vi "Universal I-V.vi"() -> ()   [LabVIEW 2021]
panel:
  in  "Tab Control 2":enum32{"V1 vs I", "V2 vs I", "V3 vs I"}(tab)=enum."V2 vs I"
  out "XY Graph":cluster{"Y":dbl[], "Y":dbl[]}[](graph)=[{"Y"=[-1.0, -0.95, -0.9, -0.85, -0.8, -0.75, -0.7, -0.6499999999999999, -0.6, -0.55, -0.5, -0.44999999999999996, -0.3999999999999999, -0.35, -0.29999999999999993, -0.25, -0.19999999999999996, -0.1499999999999999, -0.09999999999999998, -0.04999999999999993, 0.0, 0.050000000000000044, 0.10000000000000009, 0.15000000000000013, 0.20000000000000018, 0.25, 0.30000000000000004, 0.3500000000000001, 0.40000000000000013, 0.4500000000000002, 0.5, 0.55, 0.6000000000000001, 0.6500000000000001, 0.7000000000000002, 0.75, 0.8, 0.8500000000000001, 0.9000000000000001, 0.9500000000000002, 1.0, 0.9499999999999997, 0.8999999999999999, 0.8500000000000001, 0.7999999999999998, 0.75, 0.6999999999999997, 0.6499999999999999, 0.5999999999999996, 0.5499999999999998, 0.5, 0.44999999999999973, 0.3999999999999999, 0.34999999999999964, 0.2999999999999998, 0.25, 0.19999999999999973, 0.1499999999999999, 0.09999999999999964, 0.04999999999999982, 0.0, -0.050000000000000266, -0.10000000000000009, -0.15000000000000036, -0.20000000000000018, -0.25, -0.30000000000000027, -0.3500000000000001, -0.40000000000000036, -0.4500000000000002, -0.5, -0.5500000000000003, -0.6000000000000001, -0.6500000000000004, -0.7000000000000002, -0.75, -0.8000000000000003, -0.8500000000000001, -0.9000000000000004, -0.9500000000000002, -1.0], "Y"=[-1.043934004639324, -0.9887925352579463, -0.9337434547255242, -0.8776183272811331, -0.82231690582607, -0.766602837334161, -0.7120604287683167, -0.6565192233796591, -0.6008463731439775, -0.5453454129858952, -0.49006848731381447, -0.4342878186943741, -0.37878107527949273, -0.3237800120154516, -0.2679185581761966, -0.213113202761182, -0.15731677133399102, -0.10218502786401004, -0.046651896362743354, 0.00868166875831078, 0.06396663101585874, 0.11957605302530742, 0.1754465244847772, 0.23063460766105412, 0.2855722696490664, 0.3412534850248921, 0.3972359875159429, 0.4523442615679825, 0.5071052297686396, 0.5630385018551626, 0.618492497279927, 0.6741412394437152, 0.7295823751559891, 0.7846829671519501, 0.8402139260072709, 0.8957539073517712, 0.9509082828151478, 1.006347213884267, 1.0618881933858204, 1.117535728296589, 1.1727142914289796, 1.1176483875247343, 1.06164806834701, 1.006077475634131, 0.9510367142452216, 0.8955137824533387, 0.840085172731705, 0.7849945500084466, 0.7292096345678497, 0.6733065967707881, 0.6182922860635163, 0.562991828830372, 0.5072925656102947, 0.4519161573664326, 0.39629383647669314, 0.3412476911337492, 0.28535017053922246, 0.23016884332060678, 0.174690100070839, 0.1194653253729142, 0.06376416679748173, 0.008442831801321127, -0.046625501982918545, -0.10205659667499047, -0.15755560828214077, -0.2133671681974733, -0.2683102894086483, -0.3239593006796162, -0.37933857613562044, -0.4349676350135405, -0.49032180903465616, -0.5456061380270941, -0.6007304953378655, -0.656422336649383, -0.7119126845425408, -0.7676135495978567, -0.8227199032513759, -0.8778352764025348, -0.9336491430031517, -0.9893680621687002, -1.0442929042963138]}]
  out "XY Graph 2":cluster{"Y":dbl[], "Y":dbl[]}[](graph)=[{"Y"=[-1.0, -0.95, -0.9, -0.85, -0.8, -0.75, -0.7, -0.6499999999999999, -0.6, -0.55, -0.5, -0.44999999999999996, -0.3999999999999999, -0.35, -0.29999999999999993, -0.25, -0.19999999999999996, -0.1499999999999999, -0.09999999999999998, -0.04999999999999993, 0.0, 0.050000000000000044, 0.10000000000000009, 0.15000000000000013, 0.20000000000000018, 0.25, 0.30000000000000004, 0.3500000000000001, 0.40000000000000013, 0.4500000000000002, 0.5, 0.55, 0.6000000000000001, 0.6500000000000001, 0.7000000000000002, 0.75, 0.8, 0.8500000000000001, 0.9000000000000001, 0.9500000000000002, 1.0, 0.9499999999999997, 0.8999999999999999, 0.8500000000000001, 0.7999999999999998, 0.75, 0.6999999999999997, 0.6499999999999999, 0.5999999999999996, 0.5499999999999998, 0.5, 0.44999999999999973, 0.3999999999999999, 0.34999999999999964, 0.2999999999999998, 0.25, 0.19999999999999973, 0.1499999999999999, 0.09999999999999964, 0.04999999999999982, 0.0, -0.050000000000000266, -0.10000000000000009, -0.15000000000000036, -0.20000000000000018, -0.25, -0.30000000000000027, -0.3500000000000001, -0.40000000000000036, -0.4500000000000002, -0.5, -0.5500000000000003, -0.6000000000000001, -0.6500000000000004, -0.7000000000000002, -0.75, -0.8000000000000003, -0.8500000000000001, -0.9000000000000004, -0.9500000000000002, -1.0], "Y"=[-7.973435467066342e-05, -7.848190915875709e-05, -7.739362381406018e-05, -7.615855996641494e-05, -7.498368817990423e-05, -7.379658485117866e-05, -7.285829683493608e-05, -7.162612993029368e-05, -7.035244015944899e-05, -6.9300205673242e-05, -6.818649159464937e-05, -6.670261243159942e-05, -6.529115687157601e-05, -6.356811887474326e-05, -5.9102640424139045e-05, -5.872764709906027e-05, -5.877560761871314e-05, -5.8881828903913574e-05, -5.897646241257462e-05, -5.882582131725415e-05, -5.8791057987534344e-05, -5.88409498033105e-05, -5.887024112734397e-05, -5.8740522406307845e-05, -5.885028440109838e-05, -5.8752753948296464e-05, -5.6673069936635304e-05, -5.391228216692724e-05, -5.2139996114801e-05, -5.074431280106586e-05, -4.946225407402698e-05, -4.8214314911060495e-05, -4.716336794969226e-05, -4.5865536969902715e-05, -4.4784976800921104e-05, -4.3704094749110955e-05, -4.268308287607421e-05, -4.1508854845143216e-05, -4.036842449568276e-05, -3.9233788034169584e-05, -3.8167390701210644e-05, -3.9282392319388965e-05, -4.03970720545855e-05, -4.153492734254879e-05, -4.2591668193889094e-05, -4.3791968721798736e-05, -4.48506408685039e-05, -4.6003624641198825e-05, -4.713922674851109e-05, -4.8200152072876724e-05, -4.9451953828060736e-05, -5.0799998505228966e-05, -5.2078194639518314e-05, -5.3781275914848375e-05, -5.7586572989640734e-05, -5.869513694812993e-05, -5.864910772455729e-05, -5.863719806533923e-05, -5.862657593681906e-05, -5.85921344897423e-05, -5.857764976913205e-05, -5.851681394213943e-05, -5.857056835005856e-05, -5.856284316571096e-05, -5.86217476965297e-05, -5.861627569097142e-05, -5.9084293111310856e-05, -6.336501090246438e-05, -6.519620148032609e-05, -6.669263406841866e-05, -6.80049497620828e-05, -6.905171224295973e-05, -7.019536141081289e-05, -7.144426621523267e-05, -7.247944091890877e-05, -7.362148067252947e-05, -7.473197592311134e-05, -7.589847875995006e-05, -7.691369673641262e-05, -7.801260420979993e-05, -7.910668344272482e-05]}]
  out "XY Graph 3":cluster{"Y":dbl[], "Y":dbl[]}[](graph)=[{"Y"=[-1.0, -0.95, -0.9, -0.85, -0.8, -0.75, -0.7, -0.6499999999999999, -0.6, -0.55, -0.5, -0.44999999999999996, -0.3999999999999999, -0.35, -0.29999999999999993, -0.25, -0.19999999999999996, -0.1499999999999999, -0.09999999999999998, -0.04999999999999993, 0.0, 0.050000000000000044, 0.10000000000000009, 0.15000000000000013, 0.20000000000000018, 0.25, 0.30000000000000004, 0.3500000000000001, 0.40000000000000013, 0.4500000000000002, 0.5, 0.55, 0.6000000000000001, 0.6500000000000001, 0.7000000000000002, 0.75, 0.8, 0.8500000000000001, 0.9000000000000001, 0.9500000000000002, 1.0, 0.9499999999999997, 0.8999999999999999, 0.8500000000000001, 0.7999999999999998, 0.75, 0.6999999999999997, 0.6499999999999999, 0.5999999999999996, 0.5499999999999998, 0.5, 0.44999999999999973, 0.3999999999999999, 0.34999999999999964, 0.2999999999999998, 0.25, 0.19999999999999973, 0.1499999999999999, 0.09999999999999964, 0.04999999999999982, 0.0, -0.050000000000000266, -0.10000000000000009, -0.15000000000000036, -0.20000000000000018, -0.25, -0.30000000000000027, -0.3500000000000001, -0.40000000000000036, -0.4500000000000002, -0.5, -0.5500000000000003, -0.6000000000000001, -0.6500000000000004, -0.7000000000000002, -0.75, -0.8000000000000003, -0.8500000000000001, -0.9000000000000004, -0.9500000000000002, -1.0], "Y"=[0.0, 0.0, 0.0, 0.0, 0.0, 0.0, 0.0, 0.0, 0.0, 0.0, 0.0, 0.0, 0.0, 0.0, 0.0, 0.0, 0.0, 0.0, 0.0, 0.0, 0.0, 0.0, 0.0, 0.0, 0.0, 0.0, 0.0, 0.0, 0.0, 0.0, 0.0, 0.0, 0.0, 0.0, 0.0, 0.0, 0.0, 0.0, 0.0, 0.0, 0.0, 0.0, 0.0, 0.0, 0.0, 0.0, 0.0, 0.0, 0.0, 0.0, 0.0, 0.0, 0.0, 0.0, 0.0, 0.0, 0.0, 0.0, 0.0, 0.0, 0.0, 0.0, 0.0, 0.0, 0.0, 0.0, 0.0, 0.0, 0.0, 0.0, 0.0, 0.0, 0.0, 0.0, 0.0, 0.0, 0.0, 0.0, 0.0, 0.0, 0.0]}]
  in  "Voltage Offset":dbl caption="Delay Time (s)" format="%#_4f"
  in  "Wire Resistance":dbl caption="Delay Time (s)" format="%#_6f"
  in  "stop":bool
  out "Cursor measured \nResistance Ohm\ndV/dI*1M":dbl=19611.57495771106
  out "Voltage":dbl=-1.0442929042963138 format="%^#_4g"
  out "Current Applied":dbl
  in  "stop 2":bool
  out "Voltage Applied":dbl=-1.0
  in  "Tab Control":T1(tab)=enum."Scan Range"
  in  "Log I values":bool
  in  "File Name":string="Can-I"
  in  "base path":path=path "C:/Users/gyue/Box Sync/Guang Yue/data"
  out "Generated File name":string="20180723-220927-Can-I-uniIV"
  in  "I Channel control signal":enum32{"NI DAQ", "Keithley 2400"}(tab)
  in  "device in":tag="Dev1"
  in  "AO channel":tag="Dev1/ao0"
  in  "I scale NI DAQ":dbl=1.0 caption="Delay Time (s)" format="%#_5f"
  in  "Name of I Channel":string(combo)="Current uA"
  in  "samples per read V3":i32=1000
  in  "V3 Channel Read":enum32{"NI DAQ", "OFF"}(tab)=enum."OFF"
  in  "V3 scale":dbl=0.001 caption="Delay Time (s)" format="%#_4f"
  in  "AI channel V3":tag="Dev1/ai1"
  in  "Name of V3 Channel":string(combo)="Voltage V"
  in  "Name of V1 Channel":string(combo)="Current uA"
  in  "V1 Channel Read":enum32{"NI DAQ", "other"}(tab)
  in  "V1 scale":dbl=1.0 caption="Delay Time (s)" format="%#_4f"
  in  "AI channel V1":tag="Dev1/ai1"
  in  "samples per read V1":i32=500
  in  "samples per read V2":i32=500
  in  "V2 Channel Read":enum32{"NI DAQ", "OFF"}(tab)
  in  "V2 scale":dbl=0.001 caption="Delay Time (s)" format="%#_4f"
  in  "AI channel V2":tag="Dev1/ai0"
  in  "Name of V2 Channel":string(combo)="Voltage V"
  in  "True is round":bool=TRUE
  in  "Delay Time s":dbl caption="Delay Time (s)"
  in  "Step I":dbl=0.05
  in  "Start I":dbl=-1.0
  in  "End I":dbl=1.0
  in  "error in":errorcluster
  out "error out":errorcluster
  # "I uA * scale= I signal"
  # "Raw * scale= Logged Data"
  # "Raw * scale= Logged Data"
  # "Raw * scale= Logged Data"
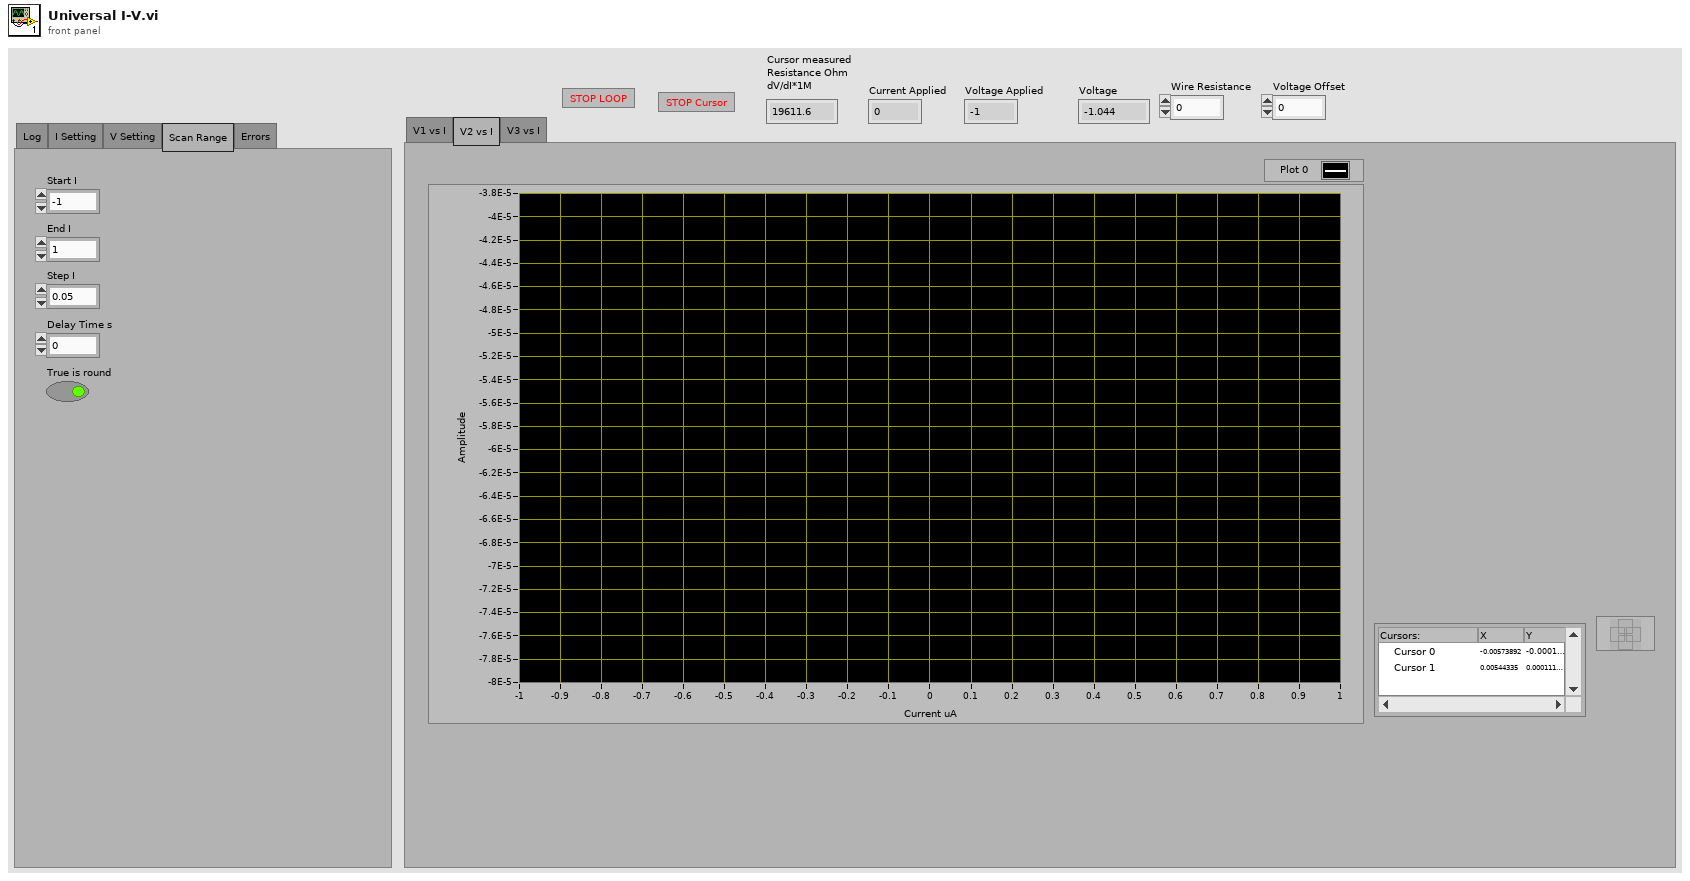
[diagram p1: front panel]
types:
  T1 = enum32{"Log", "I Setting", "V Setting", "Scan Range", "Errors"}
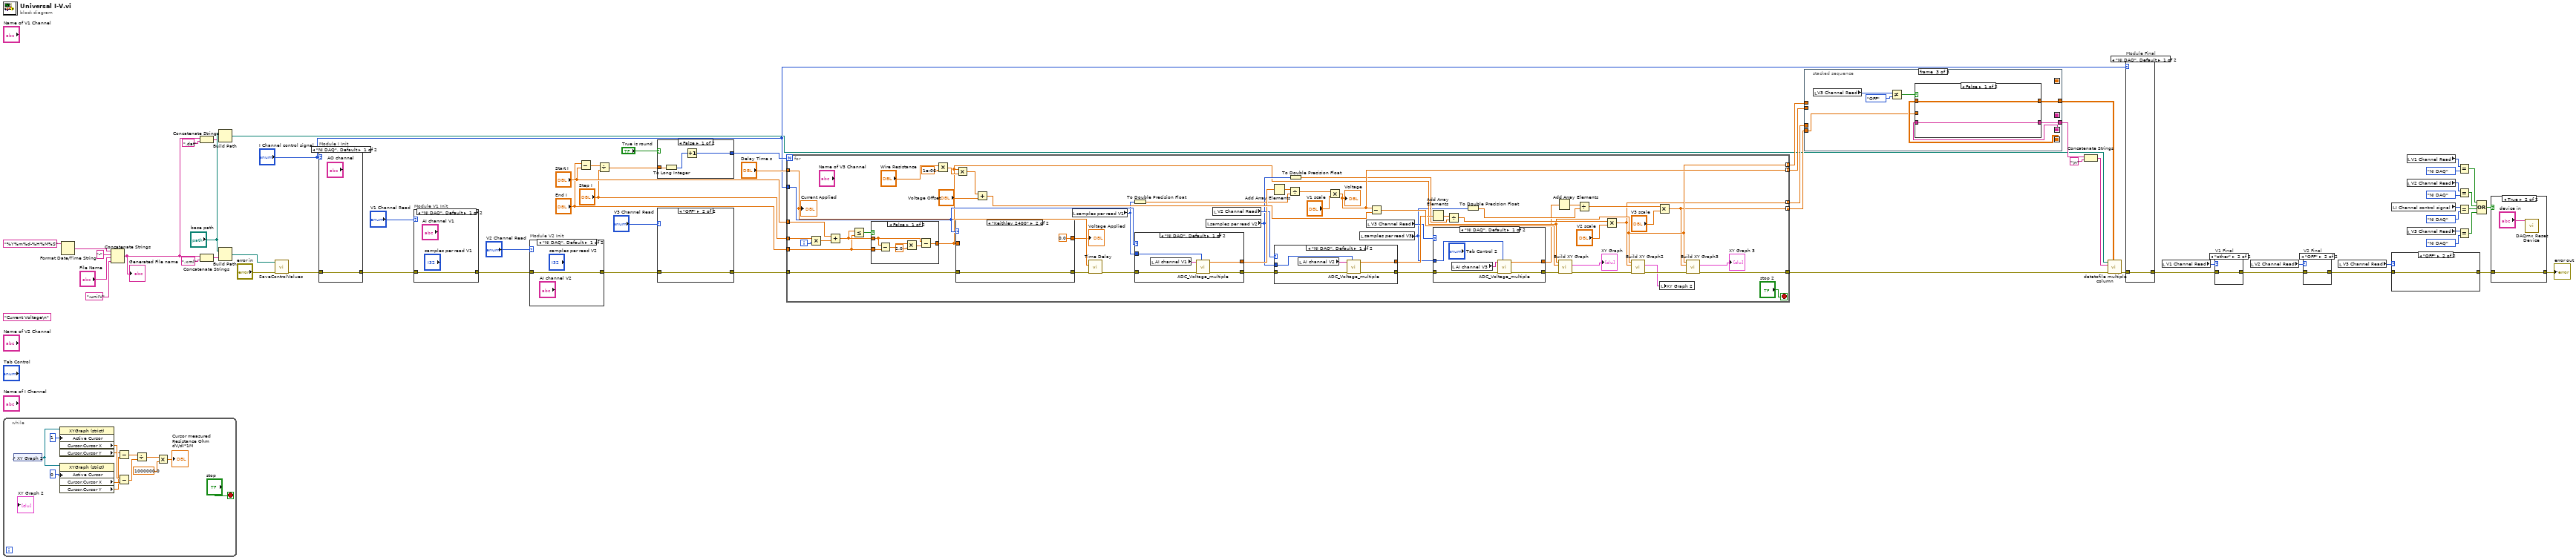
[diagram p0: block diagram]
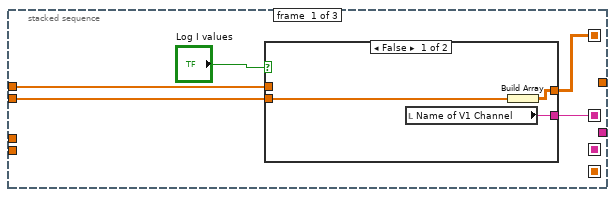
[diagram p2: hidden frame]
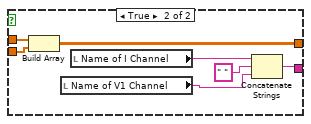
[diagram p3: hidden frame]
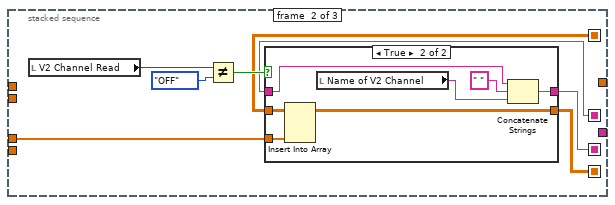
[diagram p4: hidden frame]
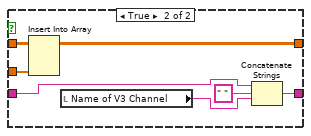
[diagram p6: hidden frame]
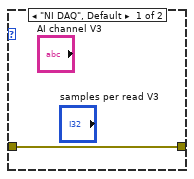
[diagram p8: hidden frame]
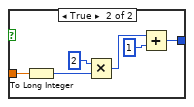
[diagram p15: hidden frame]
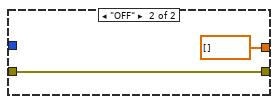
[diagram p16: hidden frame]
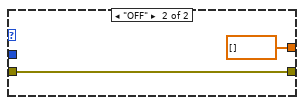
[diagram p17: hidden frame]
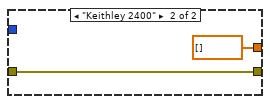
[diagram p18: hidden frame]
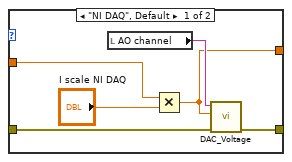
[diagram p19: hidden frame]
diagram:
  (unwired) "Current Voltage\n" ("title")
  n1 = while {
    stop <- "stop" stop-if-true
    n2 = control-ref of="XY Graph 2"() -> (w63:refnum<vi>)
    n3 = property on="Property Node" class="XYGraph (strict)"(reference=w63, "Active Cursor"=u32 1) -> ("Cursor.Cursor X"=w67:dbl, "Cursor.Cursor Y"=w65:dbl)  [unwired: 1 in, 2 out]
    n4 = property on="Property Node" class="XYGraph (strict)"(reference=w63, "Active Cursor"=u32 0) -> ("Cursor.Cursor X"=w66:dbl, "Cursor.Cursor Y"=w64:dbl)  [unwired: 1 in, 2 out]
    n5 = Subtract(x=w65, y=w64) -> (x-y=w70:dbl)
    n6 = Subtract(x=w67, y=w66) -> (x-y=w71:dbl)
    n7 = Divide(x=w70, y=w71) -> (x/y=w72:dbl)
    n8 = Multiply(x=w72, y=1000000.0) -> (x*y=→"Cursor measured \nResistance Ohm\ndV/dI*1M":dbl)
  }
  n9 = Format Date/Time String(time format string (%c)="%Y%m%d-%H%M%S") -> (date/time string=w62:string)  [unwired: 2 in]
  n10 = Concatenate Strings(w62, "-" ("string"), "File Name", "-uniIV" ("string")) -> (w54:string)
  "Generated File name" <- w54
  n11 = Concatenate Strings(w54, ".dat" ("string")) -> (w53:string)
  n12 = Concatenate Strings(w54, ".xml" ("string")) -> (w61:string)
  n13 = Build Path(base path="base path", name or relative path=w53) -> (appended path=w4:path)
  n14 = Build Path(base path="base path", name or relative path=w61) -> (appended path=w60:path)
  n15 = call "SaveControlValues.vi"("XML File Path"=w60, "error in (no error)"="error in") -> ("error out"=w50:errorcluster)  [unwired: 8 in]
  n16 = case "Module I Init" shown="\"NI DAQ\", Default" "I Channel control signal" {
    tunnel: w50 -> [w76 w77]
    tunnel: [w76 w77] -> w39
    frame "NI DAQ", Default {
    }
    frame "Keithley 2400" {
    }
  }
  n17 = case "Module V1 Init" shown="\"NI DAQ\", Default" "V1 Channel Read" {
    tunnel: w39 -> [w78 w79]
    tunnel: [w78 w79] -> w37
    frame "NI DAQ", Default {
    }
    frame "other" {
    }
  }
  n18 = case "Module V2 Init" shown="\"NI DAQ\", Default" "V2 Channel Read" {
    tunnel: w37 -> [w80 w81]
    tunnel: [w80 w81] -> w21
    frame "NI DAQ", Default {
    }
    frame "OFF" {
    }
  }
  n19 = Subtract(x="End I", y="Start I") -> (x-y=w49:dbl)
  n20 = Divide(x=w49, y="Step I") -> (x/y=w48:dbl)
  n21 = case shown="False" "True is round" {
    tunnel: w48 -> [w84 w90]
    tunnel: [w82 w88] -> w47
    frame False {
      n22 = To Long Integer(number=w84) -> (32bit integer=w83:i32)
      n23 = Increment(x=w83) -> (x+1=w82:i32)
    }
    frame True {
      n24 = To Long Integer(number=w90) -> (32bit integer=w86:i32)
      n25 = Multiply(x=2, y=w86) -> (x*y=w87:i32)
      n26 = Add(x=w87, y=1) -> (x+y=w88:i32)
    }
  }
  n27 = case shown="\"OFF\"" "V3 Channel Read" {
    tunnel: w21 -> [w91 w92]
    tunnel: [w91 w92] -> w20
    frame "NI DAQ", Default {
    }
    frame "OFF" {
    }
  }
  n28 = for {
    N: w47 -> [_]
    tunnel: "Start I" -> [w143]
    tunnel: "Step I" -> [w145]
    tunnel: "End I" -> [w140]
    tunnel: [w105] -> w12 mode=indexing
    tunnel: [w136] -> w11 mode=indexing
    tunnel: "Delay Time s" -> [w119]
    tunnel: "I Channel control signal" -> [w126]
    tunnel: w20 -> [w127]
    tunnel: [w99] -> w6
    tunnel: [w97] -> w10 mode=indexing
    tunnel: [w96] -> w9 mode=indexing
    i -> [w146]
    stop <- "stop 2" stop-if-true
    n29 = Multiply(x=w145, y=w146) -> (x*y=w144:dbl)
    n30 = Add(x=w143, y=w144) -> (x+y=w141:dbl)
    n31 = Less Or Equal?(x=w141, y=w140) -> (x <= y?=w142:bool)
    n32 = case shown="False" w142 {
      tunnel: [w179 w182] -> w105
      tunnel: w141 -> [w180 w182]
      tunnel: w140 -> [w181 _]
      frame False {
        n33 = Subtract(x=w180, y=w181) -> (x-y=w178:dbl)
        n34 = Multiply(x=w178, y=2.0) -> (x*y=w176:dbl)
        n35 = Subtract(x=w180, y=w176) -> (x-y=w179:dbl)
      }
      frame True {
      }
    }
    n36 = Multiply(x="Wire Resistance", y=1e-06) -> (x*y=w130:dbl)
    n37 = Multiply(x=w105, y=w130) -> (x*y=w134:dbl)
    n38 = case shown="\"Keithley 2400\"" w126 {
      tunnel: w105 -> [w170 _]
      tunnel: [w173 w175] -> w128
      tunnel: w127 -> [w172 w175]
      tunnel: [w168 0.0] -> w118
      frame "NI DAQ", Default {
        n39 = local read "AO channel"() -> (w171:tag)
        n40 = Multiply(x=w170, y="I scale NI DAQ") -> (x*y=w168:dbl)
        n41 = call "DAC_Voltage.vi"("error in"=w172, "Voltage"=w168, "Physical Channel(s)"=w171) -> ("error out"=w173:errorcluster)  [unwired: 8 in]
      }
      frame "Keithley 2400" {
      }
    }
    "Voltage Applied" <- w118
    n42 = Add(x=w134, y="Voltage Offset") -> (x+y=w132:dbl)
    n43 = local read "samples per read V1"() -> (w123:i32)
    n44 = call "Time Delay"("error in (no error)"=w128, "Delay Time (s)"=w119) -> ("error out"=w125:errorcluster)  [unwired: 9 in]
    n45 = To Double Precision Float(number=w123) -> (double precision float=w115:dbl)
    n46 = case shown="\"NI DAQ\", Default" w126 {
      tunnel: w123 -> [w165 _]
      tunnel: w125 -> [w164 w167]
      tunnel: [w163 w167] -> w120
      tunnel: [w162 dbl[] [] ("data")] -> w124
      frame "NI DAQ", Default {
        n47 = local read "AI channel V1"() -> (w161:tag)
        n48 = call "ADC_Voltage_multiple.vi"("samples per channel"=w165, "error in"=w164, "physical channels"=w161) -> ("error out"=w163:errorcluster, "data"=w162:dbl[])  [unwired: 7 in]
      }
      frame "Keithley 2400" {
      }
    }
    n49 = local read "samples per read V2"() -> (w114:i32)
    n50 = local read "V2 Channel Read"() -> (w121:enum32{"NI DAQ", "OFF"})
    n51 = Add Array Elements(numeric array=w124) -> (sum=w138:dbl)
    n52 = case shown="\"NI DAQ\", Default" w121 {
      tunnel: w120 -> [w158 w159]
      tunnel: w114 -> [w156 _]
      tunnel: [w155 dbl[] [] ("data")] -> w117
      tunnel: [w154 w159] -> w109
      frame "NI DAQ", Default {
        n53 = local read "AI channel V2"() -> (w157:tag)
        n54 = call "ADC_Voltage_multiple.vi"("samples per channel"=w156, "error in"=w158, "physical channels"=w157) -> ("error out"=w154:errorcluster, "data"=w155:dbl[])  [unwired: 7 in]
      }
      frame "OFF" {
      }
    }
    n55 = Divide(x=w138, y=w115) -> (x/y=w137:dbl)
    n56 = To Double Precision Float(number=w114) -> (double precision float=w113:dbl)
    n57 = Multiply(x=w137, y="V1 scale") -> (x*y=w136:dbl)
    "Voltage" <- w136
    n58 = local read "samples per read V3"() -> (w103:i32)
    n59 = local read "V3 Channel Read"() -> (w110:enum32{"NI DAQ", "OFF"})
    n60 = Subtract(x=w136, y=w132) -> (x-y=w131:dbl)
    n61 = Add Array Elements(numeric array=w117) -> (sum=w116:dbl)
    n62 = case shown="\"NI DAQ\", Default" w110 {
      tunnel: w109 -> [w150 w153]
      tunnel: w103 -> [w149 _]
      tunnel: [w148 dbl[] [] ("data")] -> w104
      tunnel: [w147 w153] -> w102
      frame "NI DAQ", Default {
        n63 = local read "AI channel V3"() -> (w151:tag)
        n64 = call "ADC_Voltage_multiple.vi"("samples per channel"=w149, "error in"=w150, "physical channels"=w151) -> ("error out"=w147:errorcluster, "data"=w148:dbl[])  [unwired: 7 in]
      }
      frame "OFF" {
      }
    }
    n65 = Divide(x=w116, y=w113) -> (x/y=w112:dbl)
    n66 = To Double Precision Float(number=w103) -> (double precision float=w107:dbl)
    n67 = Add Array Elements(numeric array=w104) -> (sum=w108:dbl)
    n68 = call "Build XY Graph"("error in (no error)"=w102, "Y Input"=w131, "X Input"=w105) -> ("error out"=w101:errorcluster, "XY Graph"=→"XY Graph":cluster{"Y":dbl[], "Y":dbl[]}[])  [unwired: 7 in]
    n69 = Divide(x=w108, y=w107) -> (x/y=w106:dbl)
    n70 = Multiply(x=w112, y="V2 scale") -> (x*y=w97:dbl)
    n71 = call "Build XY Graph2"("error in (no error)"=w101, "Y Input"=w97, "X Input"=w105) -> ("error out"=w100:errorcluster, "XY Graph"=w93:cluster{"Y":dbl[], "Y":dbl[]}[])  [unwired: 7 in]
    n72 = Multiply(x=w106, y="V3 scale") -> (x*y=w96:dbl)
    n73 = local write "XY Graph 2"(w93) -> ()
    n74 = call "Build XY Graph3"("error in (no error)"=w100, "Y Input"=w96, "X Input"=w105) -> ("error out"=w99:errorcluster, "XY Graph"=→"XY Graph 3":cluster{"Y":dbl[], "Y":dbl[]}[])  [unwired: 7 in]
    "Current Applied" <- w119
  }
  n75 = stacked-sequence {
    seq-local: [w184 _ _] -> [_ w202 _]
    seq-local: [w183 _ _] -> [_ w200 _]
    seq-local: [_ w199 _] -> [_ _ w219]
    seq-local: [_ w198 _] -> [_ _ w217]
    tunnel: w12 -> [w186 _ _]
    tunnel: w11 -> [w185 _ _]
    tunnel: w10 -> [_ w201 _]
    tunnel: w9 -> [_ _ w218]
    tunnel: [_ _ w216] -> w8
    tunnel: [_ _ w215] -> w2
    frame #0 {
      n76 = case shown="False" "Log I values" {
        tunnel: w186 -> [_ w197]
        tunnel: w185 -> [w190 w196]
        tunnel: [w189 w195] -> w184
        tunnel: [w188 w191] -> w183
        frame False {
          n77 = local read "Name of V1 Channel"() -> (w188:string)
          n78 = Build Array(w190) -> (w189:dbl[][])
        }
        frame True {
          n79 = Build Array(w197, w196) -> (w195:dbl[][])
          n80 = local read "Name of V1 Channel"() -> (w192:string)
          n81 = local read "Name of I Channel"() -> (w194:string)
          n82 = Concatenate Strings(w194, " " ("string"), w192) -> (w191:string)
        }
      }
    }
    frame #1 {
      n83 = local read "V2 Channel Read"() -> (w204:enum32{"NI DAQ", "OFF"})
      n84 = Not Equal?(x=w204, y=enum32{"NI DAQ", "OFF"}."OFF") -> (x != y?=w205:bool)
      n85 = case shown="True" w205 {
        tunnel: w202 -> [w207 w214]
        tunnel: w201 -> [_ w213]
        tunnel: w200 -> [w206 w212]
        tunnel: [w207 w209] -> w199
        tunnel: [w206 w208] -> w198
        frame False {
        }
        frame True {
          n86 = Insert Into Array(array=w214, new element=w213) -> (w209:dbl[][])  [unwired: 2 in]
          n87 = local read "Name of V2 Channel"() -> (w210:string)
          n88 = Concatenate Strings(w212, " " ("string"), w210) -> (w208:string)
        }
      }
    }
    frame #2 {
      n89 = local read "V3 Channel Read"() -> (w222:enum32{"NI DAQ", "OFF"})
      n90 = Not Equal?(x=w222, y=enum32{"NI DAQ", "OFF"}."OFF") -> (x != y?=w220:bool)
      n91 = case shown="False" w220 {
        tunnel: w219 -> [w224 w231]
        tunnel: w218 -> [_ w230]
        tunnel: w217 -> [w223 w229]
        tunnel: [w223 w226] -> w216
        tunnel: [w224 w225] -> w215
        frame False {
        }
        frame True {
          n92 = Insert Into Array(array=w231, new element=w230) -> (w225:dbl[][])  [unwired: 2 in]
          n93 = local read "Name of V3 Channel"() -> (w227:string)
          n94 = Concatenate Strings(w229, " " ("string"), w227) -> (w226:string)
        }
      }
    }
  }
  n95 = Concatenate Strings(w8, "\n" ("string")) -> (w3:string)
  n96 = call "datatofile multiple column.vi"("2D data"=w2, "error in"=w6, "title"=w3, "file path (dialog if empty)"=w4) -> ("error out"=w5:errorcluster)  [unwired: 7 in]
  n97 = case "Module Final" shown="\"NI DAQ\", Default" "I Channel control signal" {
    tunnel: w5 -> [w232 w233]
    tunnel: [w232 w233] -> w34
    frame "NI DAQ", Default {
    }
    frame "Keithley 2400" {
    }
  }
  n98 = local read "V1 Channel Read"() -> (w36:enum32{"NI DAQ", "other"})
  n99 = case "V1 Final" shown="\"other\"" w36 {
    tunnel: w34 -> [w234 w235]
    tunnel: [w234 w235] -> w33
    frame "NI DAQ", Default {
    }
    frame "other" {
    }
  }
  n100 = local read "V2 Channel Read"() -> (w35:enum32{"NI DAQ", "OFF"})
  n101 = case "V2 Final" shown="\"OFF\"" w35 {
    tunnel: w33 -> [w236 w237]
    tunnel: [w236 w237] -> w18
    frame "NI DAQ", Default {
    }
    frame "OFF" {
    }
  }
  n102 = local read "V3 Channel Read"() -> (w19:enum32{"NI DAQ", "OFF"})
  n103 = local read "I Channel control signal"() -> (w28:enum32{"NI DAQ", "Keithley 2400"})
  n104 = case shown="\"OFF\"" w19 {
    tunnel: w18 -> [w238 w239]
    tunnel: [w238 w239] -> w17
    frame "NI DAQ", Default {
    }
    frame "OFF" {
    }
  }
  n105 = local read "V1 Channel Read"() -> (w32:enum32{"NI DAQ", "other"})
  n106 = local read "V2 Channel Read"() -> (w30:enum32{"NI DAQ", "OFF"})
  n107 = local read "V3 Channel Read"() -> (w15:enum32{"NI DAQ", "OFF"})
  n108 = Equal?(x=w32, y=enum32{"NI DAQ", "other"}."NI DAQ") -> (x = y?=w26:bool)
  n109 = Equal?(x=w30, y=enum32{"NI DAQ", "OFF"}."NI DAQ") -> (x = y?=w25:bool)
  n110 = Equal?(x=w28, y=enum32{"NI DAQ", "Keithley 2400"}."NI DAQ") -> (x = y?=w24:bool)
  n111 = Equal?(x=w15, y=enum32{"NI DAQ", "OFF"}."NI DAQ") -> (x = y?=w16:bool)
  n112 = Compound Arithmetic op=OR(w26, w25, w24, w16) -> (w23:bool)
  n113 = case shown="True" w23 {
    tunnel: [w240 w241] -> w13
    tunnel: w17 -> [w240 w241]
    frame False {
    }
    frame True {
      n114 = call <vilib>:"DAQmx Reset Device.vi"("device in"="device in") -> ()  [unwired: 14 in, 1 out]
    }
  }
  "error out" <- w13
